vi "AcquireJoystickData.vi"() -> ()   [LabVIEW 2019]
uses:
  <vilib>/Utility/inputDevices.llb/joystickAcquire.vi
  <vilib>/Utility/inputDevices.llb/closeJoystick.vi
panel:
  out "direction info":T1
  out "button info":T2
  out "axis info":T3
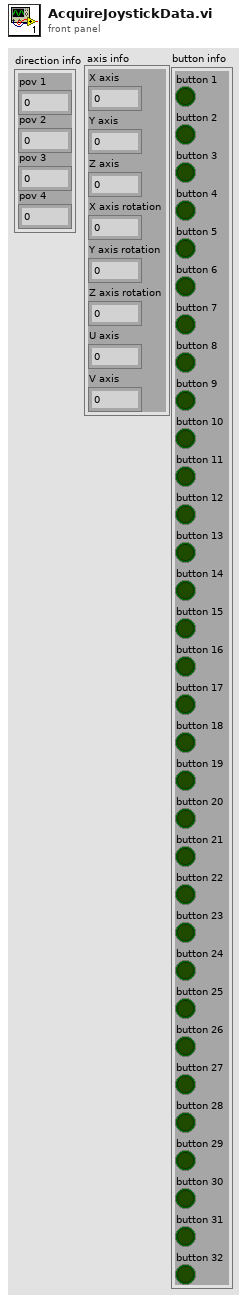
[diagram p1: front panel]
types:
  T1 = cluster{"pov 1":i32, "pov 2":i32, "pov 3":i32, "pov 4":i32}
  T2 = cluster{"button 1":bool, "button 2":bool, "button 3":bool, "button 4":bool, "button 5":bool, "button 6":bool, "button 7":bool, "button 8":bool, "button 9":bool, "button 10":bool, "button 11":bool, "button 12":bool, "button 13":bool, "button 14":bool, "button 15":bool, "button 16":bool, "button 17":bool, "button 18":bool, "button 19":bool, "button 20":bool, "button 21":bool, "button 22":bool, "button 23":bool, "button 24":bool, "button 25":bool, "button 26":bool, "button 27":bool, "button 28":bool, "button 29":bool, "button 30":bool, "button 31":bool, "button 32":bool}
  T3 = cluster{"X axis":i32, "Y axis":i32, "Z axis":i32, "X axis rotation":i32, "Y axis rotation":i32, "Z axis rotation":i32, "U axis":i32, "V axis":i32}
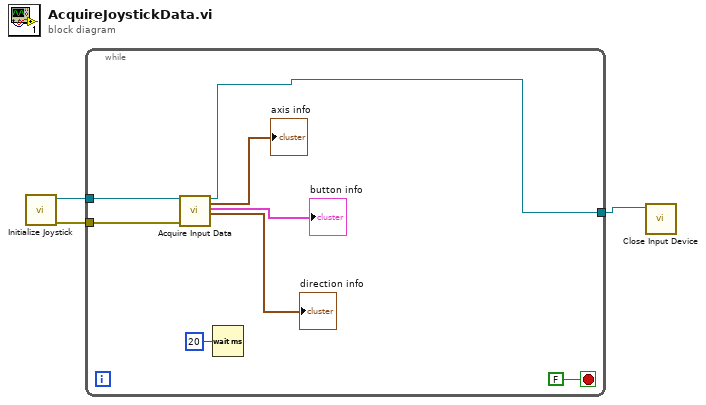
[diagram p0: block diagram]
diagram:
  n1 = call <vilib>:"Initialize Joystick.vi"() -> ("error out"=w3:errorcluster, "device ID"=w2:refnum<k1>)  [unwired: 10 in]
  n2 = while {
    tunnel: w2 -> [w10]
    tunnel: w3 -> [w5]
    tunnel: [w6] -> w1
    stop <- FALSE stop-if-true
    n3 = call-poly <vilib>:"Acquire Input Data.vi"("device ID"=w10, "error in (no error)"=w5) -> ("device ID"=w6:refnum<k1>, "axis info"=→"axis info":T3, "button info"=→"button info":T2, "direction info"=→"direction info":T1)  [unwired: 13 in, 1 out]
    n4 = Wait (ms)(milliseconds to wait=u32 20) -> ()  [unwired: 1 out]
  }
  n5 = call-poly <vilib>:"Close Input Device.vi"("device ID"=w1) -> ()  [unwired: 9 in, 1 out]
